vi "create new file.vi"(7 "template path":path, 8 "error in":errorcluster, 11 "logging path":path) -> (0 "error out":errorcluster, 3 "bin file out":refnum<file>)   [LabVIEW 2013, in "Binary datalogger runtime.lvclass"]
uses:
  Binary datalogger runtime.lvclass
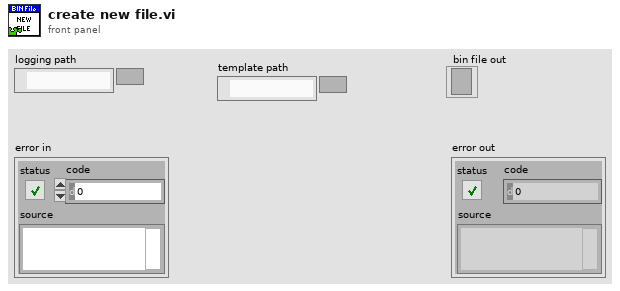
[diagram p1: front panel]
types:
  T1 = enum16{"open", "replace", "create", "open or create", "replace or create", "replace or create with confirmation"}
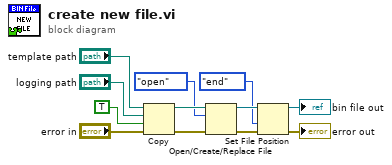
[diagram p0: block diagram]
diagram:
  n1 = Copy(8:"error in", 9:TRUE ("overwrite (F)"), 10:"logging path", 11:"template path") -> (0:w7:errorcluster, 3:w8:path)  [unwired: 1 in, 1 out]
  n2 = Open/Create/Replace File(file path (use dialog)=w8, error in=w7, operation (0:open)=T1."open") -> (refnum out=w3:refnum<file>, error out=w5:errorcluster)  [unwired: 3 in, 1 out]
  n3 = Set File Position(refnum=w3, from (0:start)=enum16{"start", "end", "current"}."end", error in=w5) -> (refnum out=→"bin file out":refnum<file>, error out=→"error out":errorcluster)  [unwired: 1 in]
